vi "Get Style Name.vi"(8 "error in (no error)":errorcluster, 11 "Style in":refnum<class "Style.lvclass">) -> (0 "error out":errorcluster, 2 "Style Name":string, 3 "Style out":refnum<class "Style.lvclass">)   [LabVIEW 2017, in "Styles.lvlib" / "Style.lvclass"]
uses:
  Style.lvclass
  Style.lvclass/Style.ctl
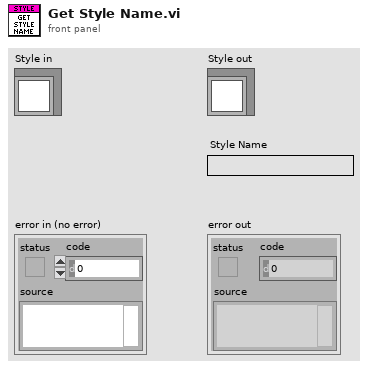
[diagram p1: front panel]
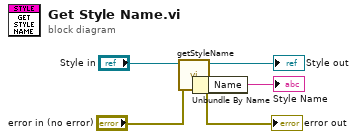
[diagram p0: block diagram]
diagram:
  n1 = call-dynamic "getStyleName.vi"("error in (no error)"="error in (no error)", "Style in"="Style in") -> ("error out"=→"error out":errorcluster, "Style out"=w2:refnum<class "Style.lvclass">)  [unwired: 7 in, 1 out]
  "Style out" <- w2
  n2 = Unbundle By Name(w2) -> ("Name"=→"Style Name":string)
